vi "APS get sscnet servo monitor data.vi"(8 "error in (no error)":errorcluster caption="错误输入（无错误）", 9 "Data_Arr":i32, 10 "Arr_Size":i32, 11 "Axis_ID":i32) -> (0 "error out":errorcluster caption="错误输出", 1 "Data_Arr out":i32, 3 "function return":i32)   [LabVIEW 2011, in "APS168.lvlib"]
doc: "I32 FNTYPE APS_get_sscnet_servo_monitor_data( I32 Axis_ID, I32 Arr_Size, I32 *Data_Arr );"
uses:
  APS168.lvlib
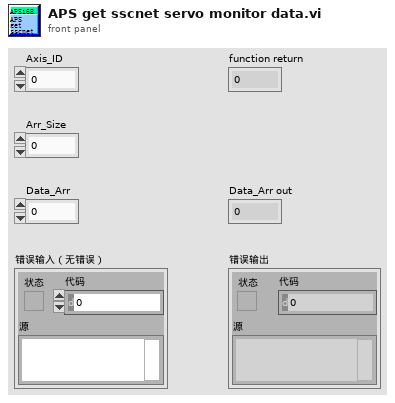
[diagram p1: front panel]
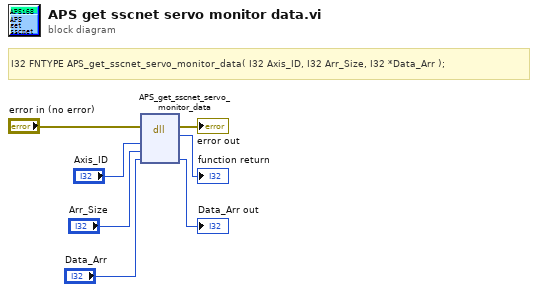
[diagram p0: block diagram]
diagram:
  # "I32 FNTYPE APS_get_sscnet_servo_monitor_data( I32 Axis_ID, I32 Arr_Size, I32 *Data_Arr );"
  n1 = dll-call lib="PTH1Labs E软件ADLINK 204CAPS_1_7_1_LIB line 连续运动204APS168.*" fn="APS_get_sscnet_servo_monitor_data"(error in="error in (no error)", "Axis_ID"="Axis_ID", "Arr_Size"="Arr_Size", "Data_Arr"="Data_Arr") -> (error out=→"error out":errorcluster, →"function return":i32, "Data_Arr"=→"Data_Arr out":i32)  [unwired: 4 in, 1 out]
